vi "WK6440B_Test.vi"(8 "error in (no error)":errorcluster, 11 "WK6440B in":refnum<class "WK6440B.lvclass">) -> (0 "error out":errorcluster, 3 "WK6440B out":refnum<class "WK6440B.lvclass">)   [LabVIEW 2018, in "WK6440B.lvclass"]
uses:
  WK6440B.lvclass
  <vilib>/Platform/TimedLoop/XDataNode/timing_clust.ctl
  <vilib>/Platform/TimedLoop/XDataNode/nitl_modes.ctl
  <vilib>/Platform/TimedLoop/XDataNode/wakeup.ctl
  InstrumentSetup.vi
  <vilib>/platform/TimedLoop/XDataNode/XDataNode.xnode
  <vilib>/Platform/TimedLoop/XDataNode/XDNodeRunTimeDep.lvlib
  InstrControl.lvclass
panel:
  out "Resistance in MOhm":dbl
  out "Capacitance in pF":dbl
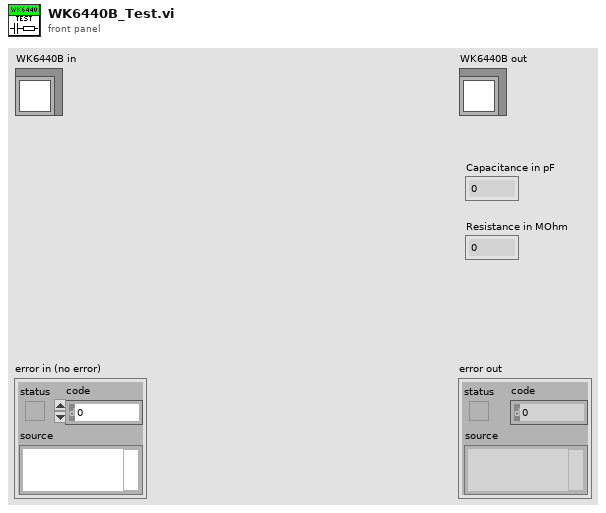
[diagram p1: front panel]
types:
  T1 = cluster{"KE 2410":cluster{"Instrument name":string, "GPIB address":string, "Instrument type":u16}, "KE 6517":cluster{"Instrument name":string, "GPIB address":string, "Instrument type":u16}, "KE 487":cluster{"Instrument name":string, "GPIB address":string, "Instrument type":u16}, "KE 487_2":cluster{"Instrument name":string, "GPIB address":string, "Instrument type":u16}, "KE 236":cluster{"Instrument name":string, "GPIB address":string, "Instrument type":u16}, "WK 6440B":cluster{"Instrument name":string, "GPIB address":string, "Instrument type":u16}, "WK 6425":cluster{"Instrument name":string, "GPIB address":string, "Instrument type":u16}, "Pickering Matrix":cluster{"Instrument name":string, "GPIB address":string, "Instrument type":u16}, "KE 2000":cluster{"Instrument name":string, "GPIB address":string, "Instrument type":u16}, "KE 2657A":cluster{"Instrument name":string, "GPIB address":string, "Instrument type":u16}, "Prague Pickering Matrix":cluster{"Instrument name":string, "GPIB address":string, "Instrument type":u16}}
  T2 = cluster{"RC Configuration":u16, "AC amplitude [V]":dbl, "AC frequency [Hz]":i32, "WK6440B":refnum<class "WK6440B.lvclass">}
  T3 = typedef "XDNodeRunTimeDep.lvlib/timing_clust.ctl" = cluster{"Expected End [f-1]":u64, "Actual End [f-1]":u64, "Finished Late? [f-1]":bool, "Expected End [i-1]":u64, "Actual End [i-1]":u64, "Finished Late? [i-1]":bool, "Expected Start [i]":u64, "Actual Start [i]":u64, "Expected Start [f]":u64, "Actual Start [f]":u64, "Source Name":string, "Structure Name":string, "Period":i64, "Deadline":i64, "Offset":i64, "Start":i64, "Priority":i32, "Timeout":i32, "Mode":T4, "Wakeup Reason":T5, "Error":errorcluster, "Source Type":string, "Secondary Source Type":string, "Global End Time":u64, "Global Start Time":u64, "Frame Duration":u64, "Iteration Duration":u64, "Assigned CPU":i32, "I/O Scan Engine Mode":u32}
  T4 = typedef "XDNodeRunTimeDep.lvlib/nitl_modes.ctl" = enum32{"No Change", "Process missed periods, maintain original phase", "Discard missed periods, maintain original phase", "Process missed periods, ignore original phase", "Discard missed periods, ignore original phase"}
  T5 = typedef "XDNodeRunTimeDep.lvlib/wakeup.ctl" = enum32{"Normal", "Aborted", "Asynchronous wakeup", "Timing source error", "Timed loop error", "Timeout"}
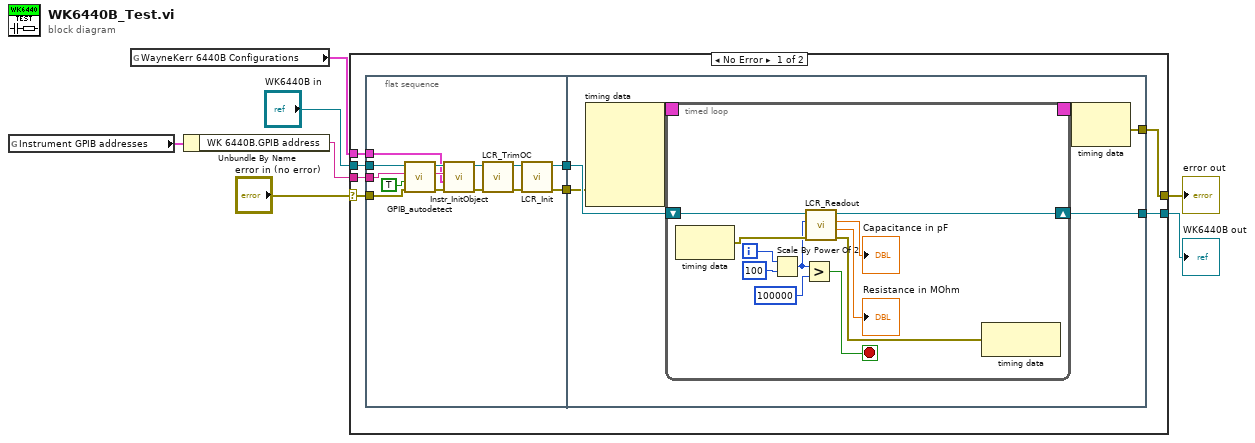
[diagram p0: block diagram]
diagram:
  n1 = global read "InstrumentSetup.vi" "Instrument GPIB addresses"() -> (w2:T1)
  n2 = global read "InstrumentSetup.vi" "WayneKerr 6440B Configurations"() -> (w3:T2)
  n3 = Unbundle By Name(w2) -> ("WK 6440B.GPIB address"=w1:string)
  n4 = case shown="No Error" "error in (no error)" {
    selector: "error in (no error)" -> [w10 w58]
    tunnel: [w15 w58] -> w6
    tunnel: [w14 w57] -> w4
    tunnel: "WK6440B in" -> [w11 w57]
    tunnel: w3 -> [w9 _]
    tunnel: w1 -> [w8 _]
    frame No Error {
      n5 = flat-sequence {
        tunnel: w11 -> [w25]
        tunnel: w10 -> [w21]
        tunnel: [w27] -> w13
        tunnel: [w26] -> w12
        tunnel: w9 -> [w18]
        tunnel: w8 -> [w17]
        tunnel: w13 -> [w32]
        tunnel: w12 -> [w30]
        tunnel: [w33] -> w15
        tunnel: [w31] -> w14
        frame #0 {
          n6 = call-dynamic "GPIB_autodetect.vi"("error in (no error)"=w21, "Verify GPIB address"=TRUE, "Instrument GPIB address in"=w17, "InstrControl in"=w25) -> ("error out"=w23:errorcluster, "Instrument GPIB address"=w22:string, "InstrControl out"=w24:refnum<class "WK6440B.lvclass">)  [unwired: 5 in]
          n7 = call-dynamic "Instr_InitObject.vi"("error in (no error)"=w23, "Instrument Configuration"=w18, "GPIB Address"=w22, "WK6440B in"=w24) -> ("error out"=w20:errorcluster, "WK6440B out"=w19:refnum<class "WK6440B.lvclass">)  [unwired: 6 in]
          n8 = call-dynamic "LCR_TrimOC.vi"("error in (no error)"=w20, "WK6440B in"=w19) -> ("error out"=w28:errorcluster, "WK6440B out"=w29:refnum<class "WK6440B.lvclass">)  [unwired: 8 in]
          n9 = call-dynamic "LCR_Init.vi"("error in (no error)"=w28, "LCRControl in"=w29) -> ("error out"=w26:errorcluster, "LCRControl out"=w27:refnum<class "WK6440B.lvclass">)  [unwired: 8 in]
        }
        frame #1 {
          n10 = node-c288(w30) -> (w35:T3)  [unwired: 4 in]
          n11 = timed-loop {
            timing: w35 -> [_]
            timing-out: [_] -> w34
            shift-right: [w38] -> w31
            shift-left: w32 -> [w39]
            i -> [w41]
            stop <- w43 stop-if-true
            n12 = node-c288() -> (w46:errorcluster)  [unwired: 1 in]
            n13 = Scale By Power Of 2(n=w41, x=100) -> (x*2^n=w40:i32)
            n14 = Greater?(x=w40, y=100000) -> (0:w43:bool)
            n15 = call-dynamic "LCR_Readout.vi"("error in (no error)"=w46, "Frequency in Hz"=w40, "WK6440B in"=w39) -> ("error out"=w45:errorcluster, "Resistance in Ohm"=→"Resistance in MOhm":dbl, "Capacitance in pF"=→"Capacitance in pF":dbl, "WK6440B out"=w38:refnum<class "WK6440B.lvclass">)  [unwired: 5 in]
            n16 = node-c288(w45) -> ()  [unwired: 1 out]
          }
          n17 = node-c288(w34) -> (w33:errorcluster)
        }
      }
    }
    frame Error {
    }
  }
  "error out" <- w6
  "WK6440B out" <- w4
